vi "Logger.Variant.CompareFiles2.vi"() -> ()   [LabVIEW 2016]
uses:
  <vilib>/Utility/miscctls.llb/LVRowAndColumnTypeDef.ctl
panel:
  in  "Station":bool
  out "sum":i16
  in  "ver":bool
  in  "All":i32(listbox)
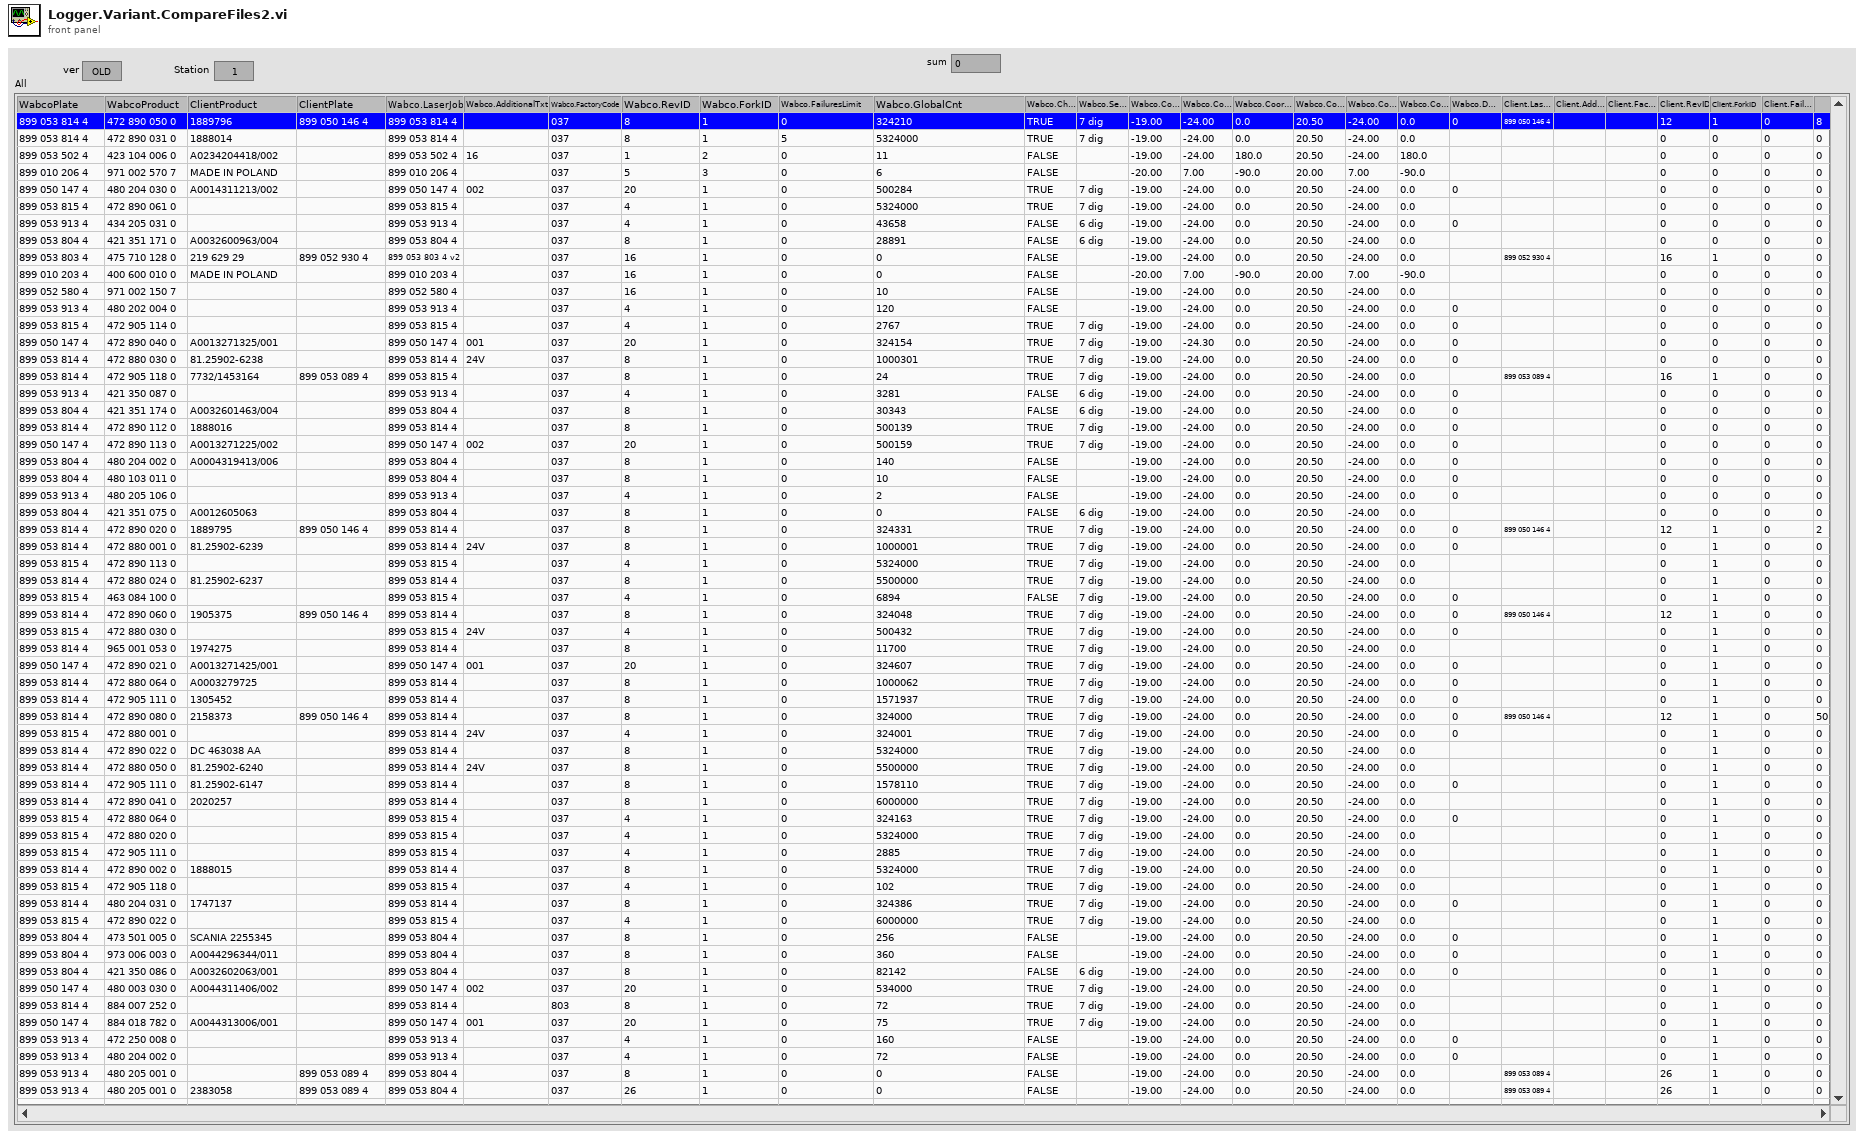
[diagram p1: front panel]
types:
  T1 = typedef "LVRowAndColumnTypeDef.ctl" = cluster{"Row":i32, "Column":i32}
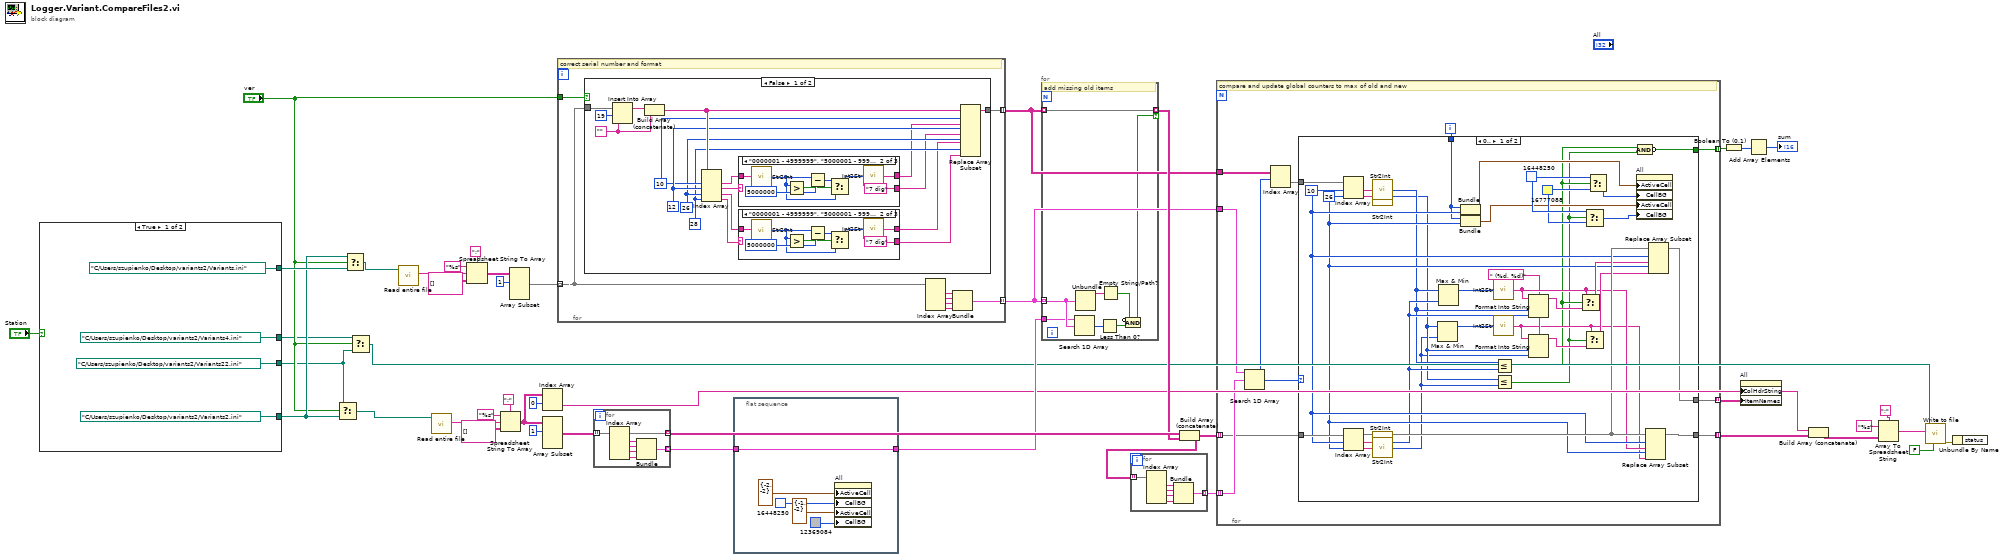
[diagram p0: block diagram]
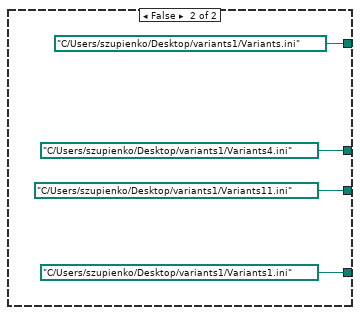
[diagram p2: hidden frame]
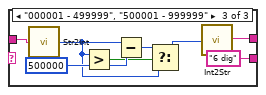
[diagram p5: hidden frame]
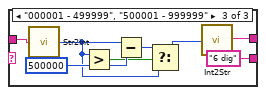
[diagram p7: hidden frame]
diagram:
  n1 = case shown="True" "Station" {
    tunnel: [path "C:/Users/szupienko/Desktop/variants2/Variants.ini" ("FilePath") path "C:/Users/szupienko/Desktop/variants1/Variants.ini" ("FilePath")] -> w16
    tunnel: [path "C:/Users/szupienko/Desktop/variants2/Variants2.ini" ("FilePath") path "C:/Users/szupienko/Desktop/variants1/Variants1.ini" ("FilePath")] -> w8
    tunnel: [path "C:/Users/szupienko/Desktop/variants2/Variants4.ini" ("FilePath") path "C:/Users/szupienko/Desktop/variants1/Variants4.ini" ("FilePath")] -> w4
    tunnel: [path "C:/Users/szupienko/Desktop/variants2/Variants22.ini" ("FilePath") path "C:/Users/szupienko/Desktop/variants1/Variants11.ini" ("FilePath")] -> w2
    frame True {
    }
    frame False {
    }
  }
  n2 = Select(t=w2, s="ver", f=w8) -> (s? t:f=w7:path)
  n3 = Select(t=w8, s="ver", f=w16) -> (s? t:f=w15:path)
  n4 = Select(t=w4, s="ver", f=w2) -> (s? t:f=w3:path)
  n5 = call "Read entire file.vi"("file"=w15) -> ("contents"=w44:string)  [unwired: 5 in, 1 out]
  n6 = call "Read entire file.vi"("file"=w7) -> ("contents"=w39:string)  [unwired: 5 in, 1 out]
  n7 = Spreadsheet String To Array(delimiter (Tab)=";", format string="%s", spreadsheet string=w44, array type (2D Dbl)=string[][] []) -> (array=w28:string[][])
  n8 = Spreadsheet String To Array(delimiter (Tab)=";", format string="%s", spreadsheet string=w39, array type (2D Dbl)=string[][] []) -> (array=w26:string[][])
  n9 = Array Subset(array=w28, index (row)=1 ("index")) -> (w34:string[][])  [unwired: 3 in]
  n10 = Index Array(array=w26, index (row)=0) -> (element=w13:string[])  [unwired: 1 in]
  n11 = Array Subset(array=w26, index (row)=1 ("index")) -> (w33:string[][])  [unwired: 3 in]
  n12 = for {
    tunnel: w34 -> [w54] mode=indexing
    tunnel: [w60] -> w23 mode=indexing
    tunnel: [w55] -> w22 mode=indexing
    tunnel: "ver" -> [w53]
    # "correct serial number and format"
    n13 = case shown="False" w53 {
      tunnel: [w73 w115] -> w60
      tunnel: w54 -> [w61 w115]
      frame False {
        w69 = 26 ("index")
        w70 = 10 ("index")
        w68 = 28 ("index")
        w74 = 12 ("index")
        w76 = ""
        n14 = Insert Into Array(array=w61, index=19, new element=w76) -> (w77:string[])
        n15 = Build Array (concatenate)(w77, w76) -> (w75:string[])
        n16 = Index Array(array=w75, index #1=w70, index #2=w74, index #3=w69, index #4=w68) -> (element #1=w64:string, element #2=w65:string, element #3=w71:string, element #4=w72:string)
        n17 = case shown="\"0000001 - 4999999\", \"5000001 - 9999999\"" w65 {
          selector: w65 -> [w80 _ _]
          tunnel: [w80 "7 dig" "6 dig"] -> w62
          tunnel: w64 -> [w79 w87 w89]
          tunnel: [w79 w81 w90] -> w63
          frame Default {
          }
          frame "0000001 - 4999999", "5000001 - 9999999" {
            w86 = 5000000 ("y")
            n18 = call "Str2Int.vi"("string"=w87) -> ("Numeric"=w83:i32)
            n19 = Greater?(x=w83, y=w86) -> (0:w85:bool)
            n20 = Subtract(x=w83, y=w86) -> (x-y=w84:i32)
            n21 = Select(t=w84, s=w85, f=w83) -> (s? t:f=w82:i32)
            n22 = call "Int2Str.vi"("Numeric"=w82) -> ("string"=w81:string)
          }
          frame "000001 - 499999", "500001 - 999999" {
            w95 = 500000 ("y")
            n23 = call "Str2Int.vi"("string"=w89) -> ("Numeric"=w92:i32)
            n24 = Greater?(x=w92, y=w95) -> (0:w94:bool)
            n25 = Subtract(x=w92, y=w95) -> (x-y=w93:i32)
            n26 = Select(t=w93, s=w94, f=w92) -> (s? t:f=w91:i32)
            n27 = call "Int2Str.vi"("Numeric"=w91) -> ("string"=w90:string)
          }
        }
        n28 = case shown="\"0000001 - 4999999\", \"5000001 - 9999999\"" w72 {
          selector: w72 -> [w98 _ _]
          tunnel: [w98 "7 dig" "6 dig"] -> w67
          tunnel: w71 -> [w97 w105 w107]
          tunnel: [w97 w99 w108] -> w66
          frame Default {
          }
          frame "0000001 - 4999999", "5000001 - 9999999" {
            w104 = 5000000 ("y")
            n29 = call "Str2Int.vi"("string"=w105) -> ("Numeric"=w101:i32)
            n30 = Greater?(x=w101, y=w104) -> (0:w103:bool)
            n31 = Subtract(x=w101, y=w104) -> (x-y=w102:i32)
            n32 = Select(t=w102, s=w103, f=w101) -> (s? t:f=w100:i32)
            n33 = call "Int2Str.vi"("Numeric"=w100) -> ("string"=w99:string)
          }
          frame "000001 - 499999", "500001 - 999999" {
            w113 = 500000 ("y")
            n34 = call "Str2Int.vi"("string"=w107) -> ("Numeric"=w110:i32)
            n35 = Greater?(x=w110, y=w113) -> (0:w112:bool)
            n36 = Subtract(x=w110, y=w113) -> (x-y=w111:i32)
            n37 = Select(t=w111, s=w112, f=w110) -> (s? t:f=w109:i32)
            n38 = call "Int2Str.vi"("Numeric"=w109) -> ("string"=w108:string)
          }
        }
        n39 = Replace Array Subset(array=w75, new element #1=w63, index #1=w70, new element #2=w62, index #2=w74, new element #3=w66, index #3=w69, new element #4=w67, index #4=w68) -> (w73:string[])
      }
      frame True {
      }
    }
    n40 = Index Array(array=w54) -> (element #1=w56:string, element #2=w57:string, element #3=w58:string, element #4=w59:string)  [unwired: 4 in]
    n41 = Bundle(w56, w57, w58, w59) -> (w55:cluster{string, string, string, string})  [unwired: 1 in]
  }
  n42 = for {
    tunnel: w33 -> [w117] mode=indexing
    tunnel: [w118] -> w18 mode=indexing
    tunnel: [w117] -> w25 mode=indexing
    n43 = Index Array(array=w117) -> (element #1=w121:string, element #2=w120:string, element #3=w119:string, element #4=w116:string)  [unwired: 4 in]
    n44 = Bundle(w121, w120, w119, w116) -> (w118:cluster{string, string, string, string})  [unwired: 1 in]
  }
  n45 = flat-sequence {
    tunnel: w18 -> [w122]
    tunnel: [w122] -> w17
    frame #0 {
      n46 = property on="All" class="MCListbox (strict)"("ActiveCell"=T1 {"Row"=-2, "Column"=-2} ("Active Cell:Active Cell"), "CellBG"=u32 16448250, "ActiveCell"=T1 {"Row"=-1, "Column"=-2} ("Active Cell:Active Cell"), "CellBG"=u32 12369084) -> ()  [unwired: 2 in, 2 out]
    }
  }
  n47 = for {
    tunnel: w22 -> [w130] mode=indexing
    tunnel: w23 -> [w128] mode=indexing
    tunnel: w17 -> [w129]
    tunnel: [w128] -> w24 mode=indexing if=w127
    # "add missing old items"
    n48 = Search 1D Array(1D array=w129, element=w130) -> (index of element=w134:i32)  [unwired: 1 in]
    n49 = Unbundle(w130) -> (w133:string)  [unwired: 3 out]
    n50 = Less Than 0?(x=w134) -> (x < 0?=w132:bool)
    n51 = Empty String/Path?(string/path=w133) -> (empty?=w131:bool)
    n52 = Compound Arithmetic op=AND(invert w131, w132) -> (w127:bool)
  }
  n53 = Build Array (concatenate)(w25, w24) -> (w21:string[][])
  n54 = for {
    tunnel: w21 -> [w136] mode=indexing
    tunnel: [w137] -> w20 mode=indexing
    n55 = Index Array(array=w136) -> (element #1=w140:string, element #2=w139:string, element #3=w138:string, element #4=w135:string)  [unwired: 4 in]
    n56 = Bundle(w140, w139, w138, w135) -> (w137:cluster{string, string, string, string})  [unwired: 1 in]
  }
  n57 = for {
    tunnel: w23 -> [w148]
    tunnel: w22 -> [w149]
    tunnel: w21 -> [w146] mode=indexing
    tunnel: w20 -> [w150] mode=indexing
    tunnel: [w144] -> w19 mode=indexing
    tunnel: [w143] -> w14 mode=indexing
    tunnel: [w141] -> w11 mode=indexing
    i -> [w142]
    # "compare and update global counters to max of old and new"
    n58 = Search 1D Array(1D array=w149, element=w150) -> (index of element=w147:i32)  [unwired: 1 in]
    n59 = Index Array(array=w148, index (row)=w147) -> (element=w145:string[])  [unwired: 1 in]
    n60 = case shown="0.." w147 {
      tunnel: w146 -> [w175 w184]
      tunnel: w145 -> [w183 _]
      tunnel: [w178 w184] -> w144
      tunnel: [w174 w184] -> w143
      tunnel: w142 -> [w170 _]
      tunnel: [w151 _] -> w141
      frame 0.. {
        w159 = " (%d, %d)" ("format string")
        w167 = u32 16777088
        w168 = u32 16448250
        w171 = 10 ("index")
        w169 = 26 ("index")
        n61 = Index Array(array=w183, index #1=w171, index #2=w169) -> (element #1=w182:string, element #2=w181:string)
        n62 = Index Array(array=w175, index #1=w171, index #2=w169) -> (element #1=w180:string, element #2=w179:string)
        n63 = call "Str2Int.vi"("string"=w182) -> ("Numeric"=w156:i32)
        n64 = call "Str2Int.vi"("string"=w181) -> ("Numeric"=w155:i32)
        n65 = call "Str2Int.vi"("string"=w180) -> ("Numeric"=w161:i32)
        n66 = call "Str2Int.vi"("string"=w179) -> ("Numeric"=w154:i32)
        n67 = Max & Min(x=w155, y=w154) -> (max(x,y)=w176:i32)  [unwired: 1 out]
        n68 = Max & Min(x=w156, y=w161) -> (max(x,y)=w177:i32)  [unwired: 1 out]
        n69 = Bundle(w170, "index"=w171) -> (w165:cluster{i32, "index":i32})  [unwired: 1 in]
        n70 = Bundle(w170, "index"=w169) -> (w164:cluster{i32, "index":i32})  [unwired: 1 in]
        n71 = call "Int2Str.vi"("Numeric"=w177) -> ("string"=w162:string)
        n72 = call "Int2Str.vi"("Numeric"=w176) -> ("string"=w158:string)
        n73 = Less Or Equal?(x=w156, y=w161) -> (x <= y?=w153:bool)
        n74 = Less Or Equal?(x=w155, y=w154) -> (x <= y?=w152:bool)
        n75 = Format Into String(format string=w159, initial string=w162, w156, w161) -> (resulting string=w160:string)  [unwired: 1 in, 1 out]
        n76 = Format Into String(format string=w159, initial string=w158, w155, w154) -> (resulting string=w157:string)  [unwired: 1 in, 1 out]
        n77 = Select(t=w162, s=w153, f=w160) -> (s? t:f=w173:string)
        n78 = Select(t=w168, s=w152, f=w167) -> (s? t:f=w163:u32)
        n79 = Select(t=w158, s=w152, f=w157) -> (s? t:f=w172:string)
        n80 = Select(t=w168, s=w153, f=w167) -> (s? t:f=w166:u32)
        n81 = property on="All" class="MCListbox (strict)"("ActiveCell"=w165, "CellBG"=w166, "ActiveCell"=w164, "CellBG"=w163) -> ()  [unwired: 2 in, 2 out]
        n82 = Compound Arithmetic op=AND(w153, w152) -> (invert w151:bool)
        n83 = Replace Array Subset(array=w175, new element #1=w162, index #1=w171, new element #2=w158, index #2=w169) -> (w174:string[])
        n84 = Replace Array Subset(array=w175, new element #1=w173, index #1=w171, new element #2=w172, index #2=w169) -> (w178:string[])
      }
      frame Default {
      }
    }
  }
  n85 = Boolean To (0,1)(Boolean=w11) -> (0, 1=w10:i16[])
  n86 = property on="All" class="MCListbox (strict)"("ColHdrString"=w13, "ItemNames"=w19) -> ()  [unwired: 2 in, 2 out]
  n87 = Add Array Elements(numeric array=w10) -> (sum=→"sum":i16)
  n88 = Build Array (concatenate)(w13, w14) -> (w12:string[][])
  n89 = Array To Spreadsheet String(delimiter (Tab)=";", array=w12, 3:"%s" ("format string")) -> (spreadsheet string=w29:string)
  n90 = call "Write to file.vi"("append (F)"=FALSE, "addition"=w29, "file"=w3) -> ("error out"=w6:errorcluster)  [unwired: 8 in]
  n91 = Unbundle By Name(w6) -> ()  [unwired: 1 out]
